vi "Vision Alignment.vi"(0 "Center of Mass X":dbl, 5 "Area":dbl, 7 "Gyro Angle":dbl, 9 "Res X":dbl, 11 "Res Y":dbl) -> (6 "Mecanum X Output":dbl, 8 "Mecanum Y Output":dbl, 10 "Rotation Output":dbl, 15 "At tote?":bool)   [LabVIEW 2014]
uses:
  <vilib>/addons/control/pid/pid.llb/PID (DBL).vi
  <vilib>/addons/control/pid/NI_PID_pid.lvlib
panel:
  in  "PID gains":T1={"proportional gain (Kc)"=0.003, "integral time (Ti, min)"=0.0, "derivative time (Td, min)"=0.0} {"derivative time (Td, min)" format="%.3f"; "integral time (Ti, min)" format="%.3f"; "proportional gain (Kc)" format="%.3f"}
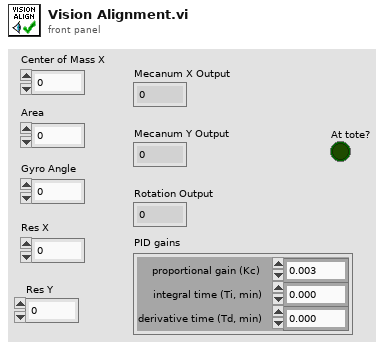
[diagram p1: front panel]
types:
  T1 = cluster{"proportional gain (Kc)":dbl, "integral time (Ti, min)":dbl, "derivative time (Td, min)":dbl}
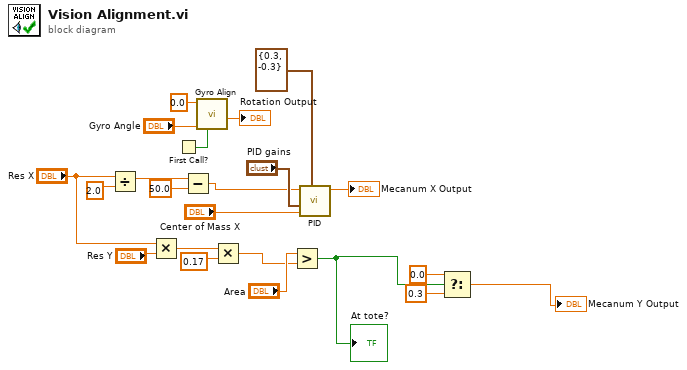
[diagram p0: block diagram]
diagram:
  n1 = Divide(x="Res X", y=2.0) -> (x/y=w4:dbl)
  n2 = Multiply(x="Res X", y="Res Y") -> (x*y=w15:dbl)
  n3 = First Call?() -> (First Call?: T/F=w1:bool)
  n4 = Subtract(x=w4, y=50.0) -> (x-y=w5:dbl)
  n5 = call "Gyro Align.vi"("Reset Setpoint"=w1, "Current Gyro Val"="Gyro Angle", "Joystick Control"=0.0) -> ("Output"=→"Rotation Output":dbl)  [unwired: 8 in]
  n6 = Multiply(x=w15, y=0.17) -> (x*y=w6:dbl)
  n7 = Greater?(x="Area", y=w6) -> (0:w11:bool)
  "At tote?" <- w11
  n8 = call-poly <vilib>:"PID.vi"("output range"=cluster{"output high":dbl, "output low":dbl} {"output high"=0.3, "output low"=-0.3}, "PID gains"="PID gains", "process variable"="Center of Mass X", "setpoint"=w5) -> ("output"=→"Mecanum X Output":dbl)  [unwired: 6 in, 1 out]
  n9 = Select(t=0.0, s=w11, f=0.3) -> (s? t:f=→"Mecanum Y Output":dbl)
